vi "Get ROI Edge ROI.vi"(8 "Error In":errorcluster, 11 "ROI Descriptor":T2 {"Contours"."Type" items=["No Selection", "Point", "Line", "Rectangle", "Oval", "Polygon", "Freehand Region", "Annulus", "Unused2", "Unused3", "Broken Line", "Freehand Line", "Rotated Rectangle"]}) -> (0 "Error Out":errorcluster, 3 "ROI Edge Descriptor":T2 {"Contours"."Type" items=["No Selection", "Point", "Line", "Rectangle", "Oval", "Polygon", "Freehand Region", "Annulus", "Unused2", "Unused3", "Broken Line", "Freehand Line", "Rotated Rectangle"]})   [LabVIEW 2021, in "Image.lvlib"]
uses:
  <vilib>/vision/Image Controls.llb/IMAQ Image.ctl
  Image ROI Type.ctl
  Image.lvlib
  <vilib>/vision/NI_Vision_Development_Module.lvlib
panel:
  in  "ROI Mask Image":T1
  in  "Image Model":T1
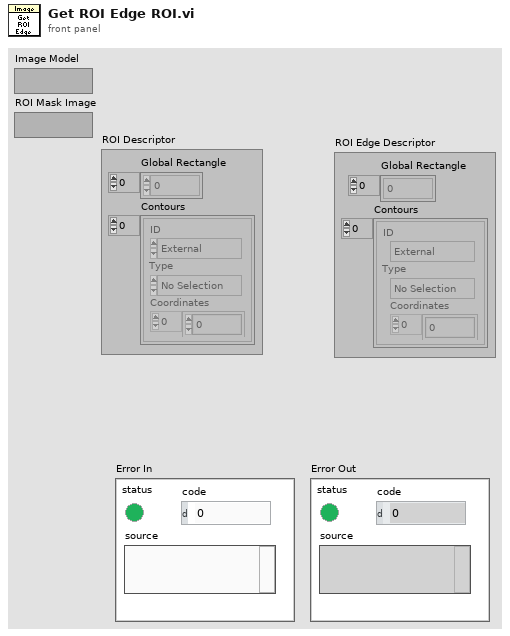
[diagram p1: front panel]
types:
  T1 = typedef "IMAQ Image.ctl" = refnum<image>
  T2 = typedef "ROI Descriptor" = cluster{"Global Rectangle":i32[], "Contours":cluster{"ID":enum32{"External", "Internal"}, "Type":u32, "Coordinates":i32[]}[]}
  T3 = typedef "Image.lvlib/Image ROI Type.ctl" = enum16{"No Selection", "Point", "Line", "Rectangle", "Oval", "Polygon", "Freehand Region", "Annulus", "Unused2", "Unused3", "Broken Line", "Freehand Line", "Rotated Rectangle"}
  T4 = cluster{"ID":enum32{"External", "Internal"}, "Type":u32, "Coordinates":i32[]}[]
  T5 = cluster{"ID":enum32{"External", "Internal"}, "Type":u32, "Coordinates":i32[]}
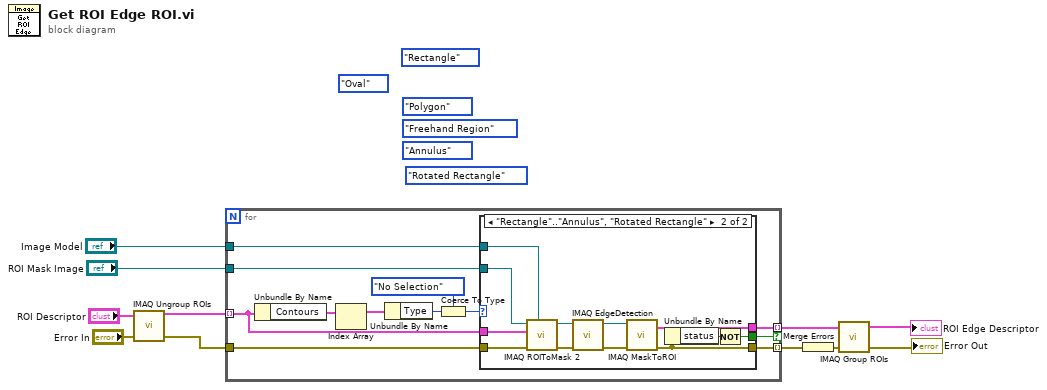
[diagram p0: block diagram]
diagram:
  (unwired) Image_ROI_Type."Rotated Rectangle" ("ROI Type")
  (unwired) Image_ROI_Type."Annulus" ("ROI Type")
  (unwired) Image_ROI_Type."Freehand Region" ("ROI Type")
  (unwired) Image_ROI_Type."Polygon" ("ROI Type")
  (unwired) Image_ROI_Type."Oval" ("ROI Type")
  (unwired) Image_ROI_Type."Rectangle" ("ROI Type")
  n1 = call "IMAQ Ungroup ROIs"("error in (no error)"="Error In", "ROI Descriptor"="ROI Descriptor") -> ("error out"=w8:errorcluster, "ROI Descriptors out"=w10:T2[])  [unwired: 2 in]
  n2 = for {
    tunnel: w10 -> [w18] mode=indexing
    tunnel: w8 -> [w17]
    tunnel: [w16] -> w6 mode=indexing
    tunnel: [w15] -> w7 mode=indexing if=w14
    tunnel: "Image Model" -> [w13]
    tunnel: "ROI Mask Image" -> [w12]
    n3 = Unbundle By Name(w18) -> ("Contours"=w23:T4)
    n4 = Index Array(array=w23) -> (element=w20:T5)  [unwired: 1 in]
    n5 = Unbundle By Name(w20) -> ("Type"=w19:u32)
    n6 = Coerce To Type(0:w19, 1:Image_ROI_Type."No Selection" ("ROI Type")) -> (2:w22:T3)
    n7 = case shown="\"Rectangle\"..\"Annulus\", \"Rotated Rectangle\"" w22 {
      tunnel: w18 -> [_ w36]
      tunnel: w17 -> [w24 w35]
      tunnel: [w24 w29] -> w16
      tunnel: [_ w30] -> w15
      tunnel: [_ w27] -> w14
      tunnel: w13 -> [_ w26]
      tunnel: w12 -> [_ w25]
      frame "No Selection", Default {
      }
      frame "Rectangle".."Annulus", "Rotated Rectangle" {
        n8 = call "IMAQ ROIToMask 2"("Image Model"=w26, "error in (no error)"=w35, "ROI Descriptor"=w36, "Image"=w25) -> ("error out"=w34:errorcluster, "Image Out"=w33:T1)  [unwired: 5 in, 1 out]
        n9 = call "IMAQ EdgeDetection"("error in (no error)"=w34, "Image Src"=w33) -> ("error out"=w32:errorcluster, "Image Dst Out"=w31:T1)  [unwired: 8 in]
        n10 = call "IMAQ MaskToROI"("Image"=w31, "error in (no error)"=w32) -> ("ROI Descriptor"=w30:T2, "error out"=w29:errorcluster)  [unwired: 5 in, 1 out]
        n11 = Unbundle By Name(w29) -> ("status"=w28:bool)
        n12 = Not(x=w28) -> (.not. x?=w27:bool)
      }
    }
  }
  n13 = Merge Errors(w6) -> (w5:errorcluster)
  n14 = call "IMAQ Group ROIs"("error in (no error)"=w5, "ROI Descriptors"=w7) -> ("error out"=→"Error Out":errorcluster, "ROI Descriptor out"=→"ROI Edge Descriptor":T2)  [unwired: 2 in]
